vi "generate_error.vi"(6 "show call chain? (T)":bool=TRUE, 8 "error in (no error)":errorcluster, 10 "Data":variant, 11 "error":T1) -> (0 "error out":errorcluster)   [LabVIEW 2015, in "lv-bin-7zip.lvlib"]
uses:
  lv-bin-7zip.lvlib
  _controls/error.ctl
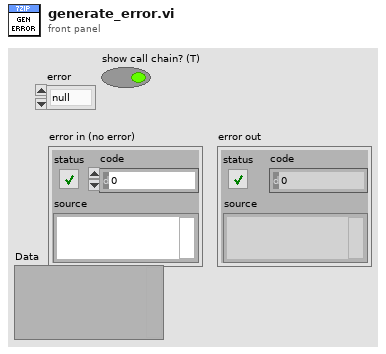
[diagram p1: front panel]
types:
  T1 = typedef "lv-bin-7zip.lvlib/error.ctl" = enum16{"null", "exe_x86_missing", "exe_x64_missing", "7za_x86_missing", "7za_x64_missing", "7zxa_x86_missing", "7zxa_x64_missing", "7zS.sfx_missing"}
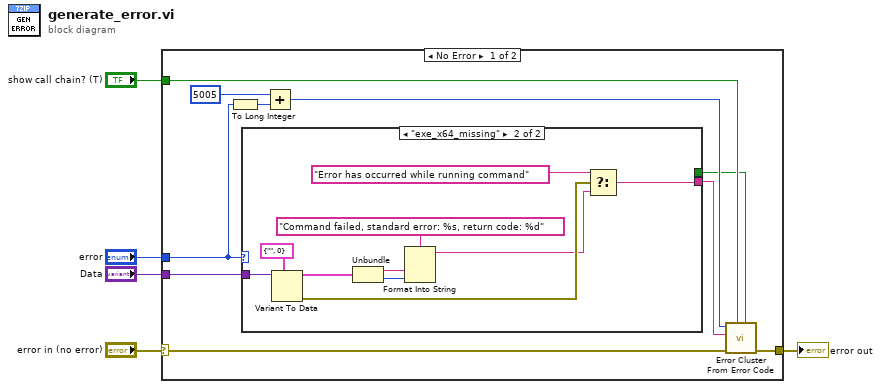
[diagram p0: block diagram]
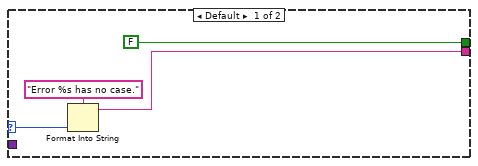
[diagram p2: hidden frame]
diagram:
  n1 = case shown="No Error" "error in (no error)" {
    selector: "error in (no error)" -> [w6 w30]
    tunnel: "Data" -> [w15 _]
    tunnel: [w14 w30] -> w3
    tunnel: "error" -> [w12 _]
    tunnel: "show call chain? (T)" -> [w8 _]
    frame No Error {
      n2 = To Long Integer(number=w12) -> (32bit integer=w11:i32)
      n3 = case shown="\"exe_x64_missing\"" w12 {
        selector: w12 -> [w18 _]
        tunnel: w15 -> [_ w29]
        tunnel: [w17 w21] -> w9
        tunnel: [FALSE _] -> w7
        frame Default {
          n4 = Format Into String(format string="Error %s has no case.", w18) -> (resulting string=w17:string)  [unwired: 2 in, 1 out]
        }
        frame "exe_x64_missing" {
          n5 = Variant To Data(type=cluster{string, "return code":i32} {"", "return code"=0} ("cluster"), Variant=w29) -> (data=w27:cluster{string, "return code":i32}, error out=w26:errorcluster)  [unwired: 1 in]
          n6 = Unbundle(w27) -> (w25:string, "return code"=w24:i32)
          n7 = Format Into String(format string="Command failed, standard error: %s, return code: %d", w25, w24) -> (resulting string=w23:string)  [unwired: 2 in, 1 out]
          n8 = Select(t="Error has occurred while running command", s=w26, f=w23) -> (s? t:f=w21:string)
        }
      }
      n9 = Add(x=5005, y=w11) -> (x+y=w10:i32)
      n10 = call <vilib>:"Error Cluster From Error Code.vi"("is warning? (False)"=w7, "show call chain? (False)"=w8, "error in (no error)"=w6, "error message (\"\")"=w9, "error code (0)"=w10) -> ("error out"=w14:errorcluster)  [unwired: 4 in]
    }
    frame Error {
    }
  }
  "error out" <- w3
